vi "IHL_Inspect-Start Helper.vi"(7 "Encoder Cnt":i32, 8 "error in (no error)":errorcluster, 9 "MaxSamples":i32, 10 "PosToEndScan":i32, 11 "EventLog in":refnum<class "EventLog.lvclass">) -> (0 "error out":errorcluster, 1 "Success":bool, 2 "data value reference":refnum<data-value>, 3 "Block Cnt notifier out":refnum<notifier>)   [LabVIEW 2015, in "Tool Module.lvlib"]
uses:
  Tool Module.lvlib
  Event Logger Library/Event Log/EventLog.lvclass
  _HS Data Stream Params Cluster--typedef.ctl
  _HS Data Stream SM enum--typedef.ctl
  ToolModGLOB.vi
  Tool Config/Tool Cfg.lvlib
  Tool Interface/Tool Interface.lvlib
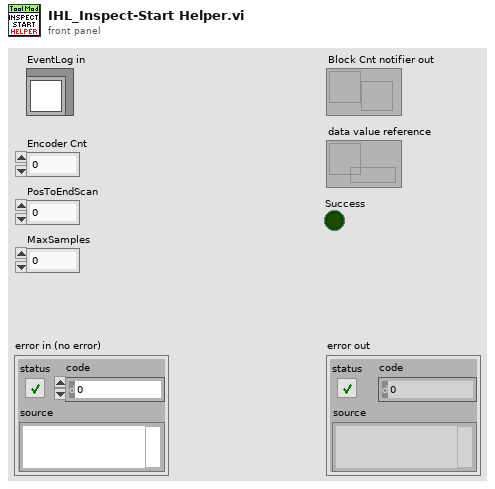
[diagram p1: front panel]
types:
  T1 = typedef "Tool Module.lvlib/_HS Data Stream SM enum--typedef.ctl" = enum16{"Idle", "Receive HS Data", "Close Connection"}
  T2 = typedef "Tool Module.lvlib/_HS Data Stream Params Cluster--typedef.ctl" = cluster{"Raw Data Stream Loop cmd":T1, "Data Array DVR ref":refnum<data-value>, "Sample Data notifier":refnum<notifier>, "Block Count Notifier":refnum<notifier>}
  T3 = typedef "Tool Cfg.lvlib/_Tool Operation Config Cluster--typedef.ctl" = cluster{"Use Tool Cfg":bool, "Use Tool Cal":bool, "Fake Data?":bool, "Mode":i16, "Array Subset Length":i16, "nArrays to Read":i16, "Full Array Read Length":i16, "nSubarrays/Sensor":i16}
  T4 = typedef "_Data Stream Fmt Params Cluster--typedef.ctl" = cluster{"Samples per Block":i32, "Raw Data Status Len":i32, "Fltr Data Status Len":i32}
  T5 = typedef "Tool Module.lvlib/_Loop Ctrl Notifiers Cluster--typedef.ctl" = cluster{"Raw Stream Ctrl":refnum<notifier>}
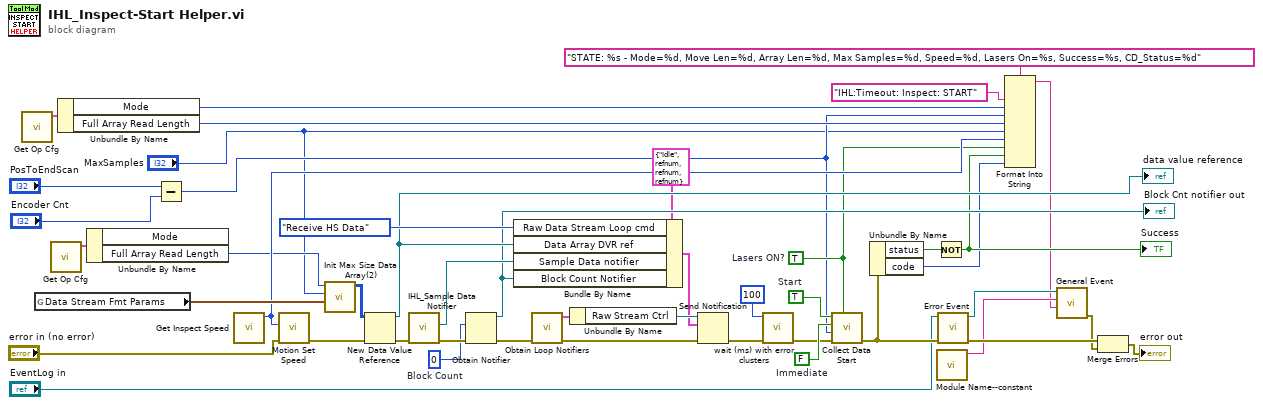
[diagram p0: block diagram]
diagram:
  w26 = FALSE  # Immediate
  w25 = TRUE  # Start
  w30 = u32 0  # Block Count
  w16 = TRUE  # Lasers ON?
  n1 = call "Get Op Cfg.vi"() -> ("Tool Operation Config"=w41:T3)  [unwired: 11 in]
  n2 = global read "ToolModGLOB.vi" "Data Stream Fmt Params"() -> (w38:T4)
  n3 = call "Get Op Cfg.vi"() -> ("Tool Operation Config"=w3:T3)  [unwired: 11 in]
  n4 = Unbundle By Name(w41) -> ("Mode"=w9:i16, "Full Array Read Length"=w8:i16)
  n5 = Unbundle By Name(w3) -> ("Full Array Read Length"=w2:i16)  [unwired: 1 out]
  n6 = Subtract(x="PosToEndScan", y="Encoder Cnt") -> (x-y=w7:i32)
  n7 = call "Get Inspect Speed.vi"() -> ("Inspect Speed"=w17:u16)  [unwired: 11 in]
  n8 = call "Motion Set Speed.vi"("error in (no error)"="error in (no error)", "Speed"=w17) -> ("error out"=w36:errorcluster)  [unwired: 9 in]
  n9 = call "Init Max Size Data Array(2).vi"("Data Stream Fmt Params"=w38, "Max Samples"="MaxSamples", "Array Length"=w2) -> ("initialized array"=w37:u32[][])  [unwired: 8 in]
  n10 = New Data Value Reference(data value=w37, error in=w36) -> (data value reference=w44:refnum<data-value>, error out=w29:errorcluster)
  "data value reference" <- w44
  n11 = call "IHL_Sample Data Notifier.vi"("error in (no error)"=w29) -> ("error out"=w42:errorcluster, "Sample Data notifier out"=w45:refnum<notifier>)  [unwired: 9 in]
  n12 = Obtain Notifier(notification data type=w30, error in (no error)=w42) -> (notifier out=w43:refnum<notifier>, error out=w23:errorcluster)  [unwired: 2 in, 1 out]
  "Block Cnt notifier out" <- w43
  n13 = Bundle By Name(cluster=T2 {"Raw Data Stream Loop cmd"=enum."Idle", "Data Array DVR ref"=refnum, "Sample Data notifier"=refnum, "Block Count Notifier"=refnum} ("_HS Data Stream Params Cluster--typedef"), "Raw Data Stream Loop cmd"=_HS_Data_Stream_SM_enum--typedef."Receive HS Data" ("HS Data Stream SM enum"), "Data Array DVR ref"=w44, "Sample Data notifier"=w45, "Block Count Notifier"=w43) -> (w27:T2)
  n14 = call "Obtain Loop Notifiers.vi"("error in (no error)"=w23) -> ("error out"=w28:errorcluster, "Loop Ctrl Notifiers Cluster"=w32:T5)  [unwired: 9 in]
  n15 = Unbundle By Name(w32) -> ("Raw Stream Ctrl"=w31:refnum<notifier>)
  n16 = Send Notification(notification=w27, notifier=w31, error in (no error)=w28) -> (error out=w6:errorcluster)  [unwired: 1 out]
  n17 = call "wait (ms) with error clusters.vi"("error in (no error)"=w6, "milliseconds to wait"=u32 100 ("milliseconds")) -> ("error out"=w5:errorcluster)  [unwired: 9 in]
  n18 = call "Collect Data Start.vi"("Lasers ON?"=w16, "error in (no error)"=w5, "Length"=w7, "Immediate"=w26, "Start"=w25) -> ("error out"=w24:errorcluster)  [unwired: 6 in]
  n19 = Unbundle By Name(w24) -> ("status"=w11:bool, "code"=w14:i32)
  n20 = Not(x=w11) -> (.not. x?=w15:bool)
  "Success" <- w15
  n21 = call "Module Name--constant.vi"() -> ("Module Name"=w19:string)  [unwired: 11 in]
  n22 = call "Error Event.vi"("error in (no error)"=w24, "EventLog ref"="EventLog in") -> ("error out"=w34:errorcluster, "EventLog ref"=w20:refnum<class "EventLog.lvclass">)  [unwired: 8 in]
  n23 = Format Into String(format string="STATE: %s - Mode=%d, Move Len=%d, Array Len=%d, Max Samples=%d, Speed=%d, Lasers On=%s, Success=%s, CD_Status=%d", "IHL:Timeout: Inspect: START", w9, w7, w8, "MaxSamples", w17, w16, w15, w14) -> (resulting string=w12:string)  [unwired: 2 in, 1 out]
  n24 = call "General Event.vi"("Event Description"=w12, "Event Name"=w19, "EventLog ref"=w20) -> ("error out"=w21:errorcluster)  [unwired: 7 in, 1 out]
  n25 = Merge Errors(w34, w21) -> (→"error out":errorcluster)
